vi "Velocity_flt.vi"() -> (1 "VZ":dbl, 2 "VY":dbl, 3 "VX":dbl)   [LabVIEW 2017]
uses:
  Program Files/National Instruments/LabVIEW 2019/user.lib/HapticSTM/HapticSTM.lvlib
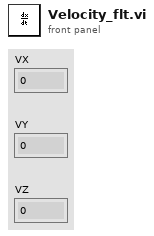
[diagram p1: front panel]
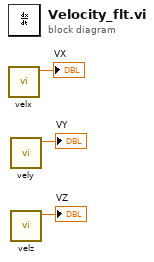
[diagram p0: block diagram]
diagram:
  n1 = call "velx.vi"() -> ("function return"=→"VX":dbl)  [unwired: 11 in]
  n2 = call "vely.vi"() -> ("function return"=→"VY":dbl)  [unwired: 11 in]
  n3 = call "velz.vi"() -> ("function return"=→"VZ":dbl)  [unwired: 11 in]
